vi "Wait for Process Running Event.vi"(8 "error in (no error)":errorcluster) -> (0 "error out":errorcluster, 3 "Panel Running?":bool)   [LabVIEW 2020, in "Generic Plugin.lvclass"]
doc: "Waits for a message with the specified command, ignoring all other messages. This is a blocking VI."
uses:
  Generic Plugin.lvclass
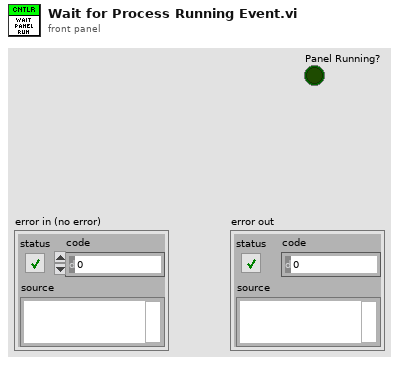
[diagram p1: front panel]
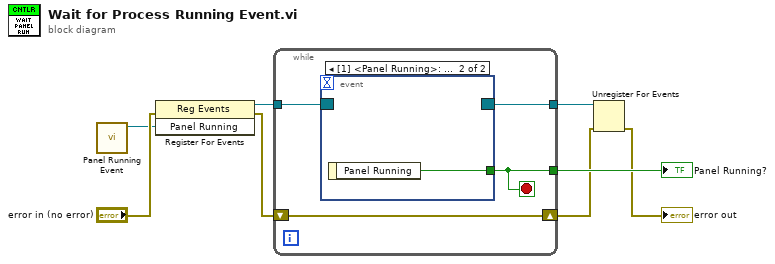
[diagram p0: block diagram]
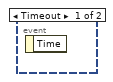
[diagram p2: hidden frame]
diagram:
  n1 = call "Panel Running Event.vi"() -> ("Panel Running"=w1:refnum<user-event>)  [unwired: 11 in]
  n2 = register-events(error in="error in (no error)", w1) -> (reference out=w8:refnum<event-registration>, error out=w2:errorcluster)  [unwired: 1 in]
  n3 = while {
    shift-right: [w12] -> w5
    shift-left: w2 -> [w12]
    tunnel: w8 -> [w11]
    tunnel: [w10] -> w7
    tunnel: [w9] -> w6
    stop <- w9 stop-if-true
    n4 = event shown="[1] <Panel Running>: User Event" {
      selector: w11 -> [_ _]
      dyn-events: [_ _] -> w10
      timeout: _ -> [_ _]
      tunnel: [_ w13] -> w9
      event Timeout {
        n5 = event-data() -> ()  [unwired: 1 in, 1 out]
      }
      event User Event {
        n6 = event-data() -> ("Panel Running"=w13:bool)  [unwired: 1 in]
      }
    }
  }
  "Panel Running?" <- w6
  n7 = Unregister For Events(event registration refnum=w7, error in=w5) -> (error out=→"error out":errorcluster)
